vi "Set Name.vi"(8 "error in (no error)":errorcluster, 10 "ID(\"\")":string, 11 "MemberInfo in":refnum<class "Information.lvclass">) -> (0 "error out":errorcluster, 3 "MemberInfo out":refnum<class "Information.lvclass">)   [LabVIEW 2015, in "Member_Actor.lvlib" / "Information.lvclass"]
uses:
  Information.lvclass
  Information.lvclass/Information.ctl
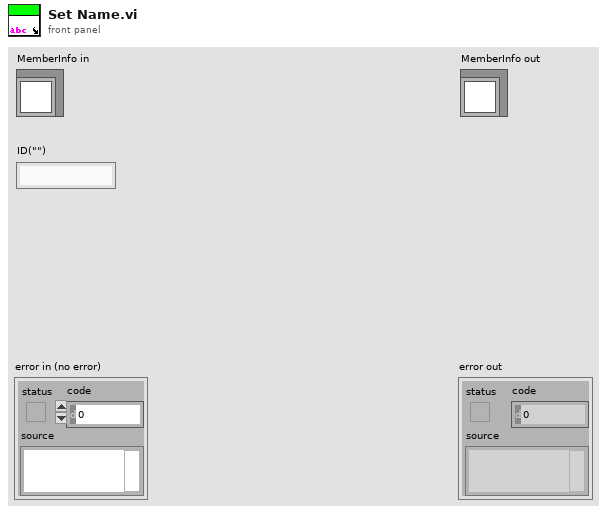
[diagram p1: front panel]
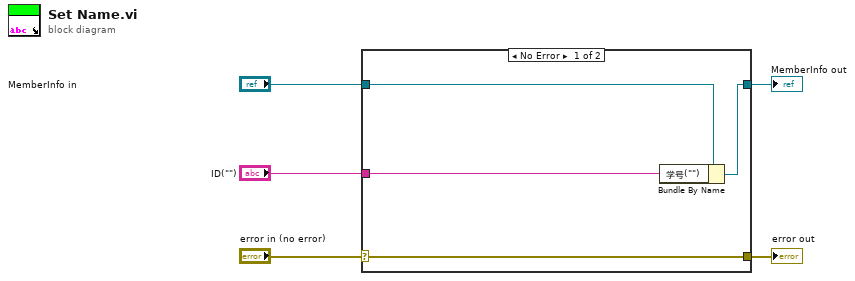
[diagram p0: block diagram]
diagram:
  n1 = case shown="No Error" "error in (no error)" {
    selector: "error in (no error)" -> [w9 w10]
    tunnel: [w9 w10] -> w4
    tunnel: [w7 w11] -> w2
    tunnel: "MemberInfo in" -> [w8 w11]
    tunnel: "ID(\"\")" -> [w6 _]
    frame No Error {
      n2 = Bundle By Name(cluster=w8, "学号(\"\")"=w6) -> (w7:refnum<class "Information.lvclass">)
    }
    frame Error {
    }
  }
  "error out" <- w4
  "MemberInfo out" <- w2
